vi "Structure Error Handle.vi"(7 "Two Selection(F)":bool, 8 "error in":errorcluster) -> (0 "error out":errorcluster)   [LabVIEW 2018]
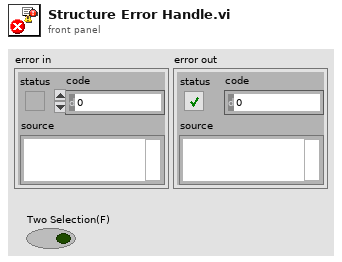
[diagram p1: front panel]
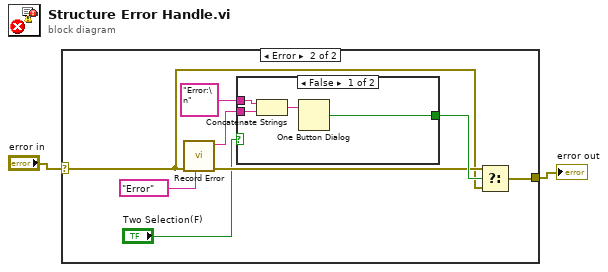
[diagram p0: block diagram]
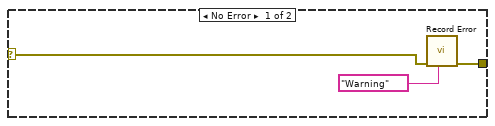
[diagram p2: hidden frame]
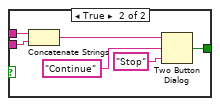
[diagram p3: hidden frame]
diagram:
  n1 = case shown="Error" "error in" {
    selector: "error in" -> [w5 w8]
    tunnel: [w3 w7] -> w1
    frame No Error {
      n2 = call "Record Error.vi"("Type"="Warning", "error in"=w5) -> ("error out"=w3:errorcluster)  [unwired: 8 in, 1 out]
    }
    frame Error {
      n3 = call "Record Error.vi"("Type"="Error", "error in"=w8) -> ("error out"=w9:errorcluster, "Error string"=w11:string)  [unwired: 8 in]
      n4 = case shown="False" "Two Selection(F)" {
        tunnel: "Error:\n" ("string") -> [w16 w20]
        tunnel: w11 -> [w15 w19]
        tunnel: [w17 w18] -> w10
        frame False {
          n5 = Concatenate Strings(w16, w15) -> (w14:string)
          n6 = One Button Dialog(message=w14) -> (true=w17:bool)  [unwired: 1 in]
        }
        frame True {
          n7 = Concatenate Strings(w20, w19) -> (w21:string)
          n8 = Two Button Dialog(message=w21, 1:"Stop" ("F button name (\"Cancel\")"), 2:"Continue" ("T button name (\"OK\")")) -> (T button?=w18:bool)
        }
      }
      n9 = Select(t=w9, s=w10, f=w8) -> (s? t:f=w7:errorcluster)
    }
  }
  "error out" <- w1
